vi "MainTypeClassic.vi"() -> ()   [LabVIEW 2014]
panel:
  in  "ButtonC":bool
  in  "ButtonB":bool
  in  "ButtonA":bool
  out "NowTime":timestamp
  out "MsgString":string
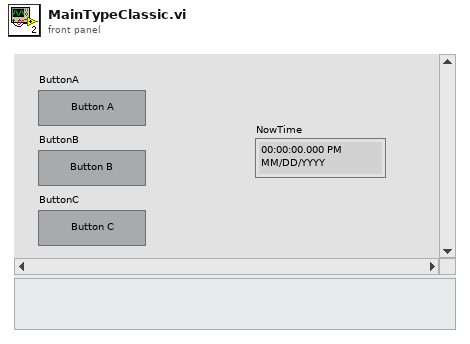
[diagram p1: front panel]
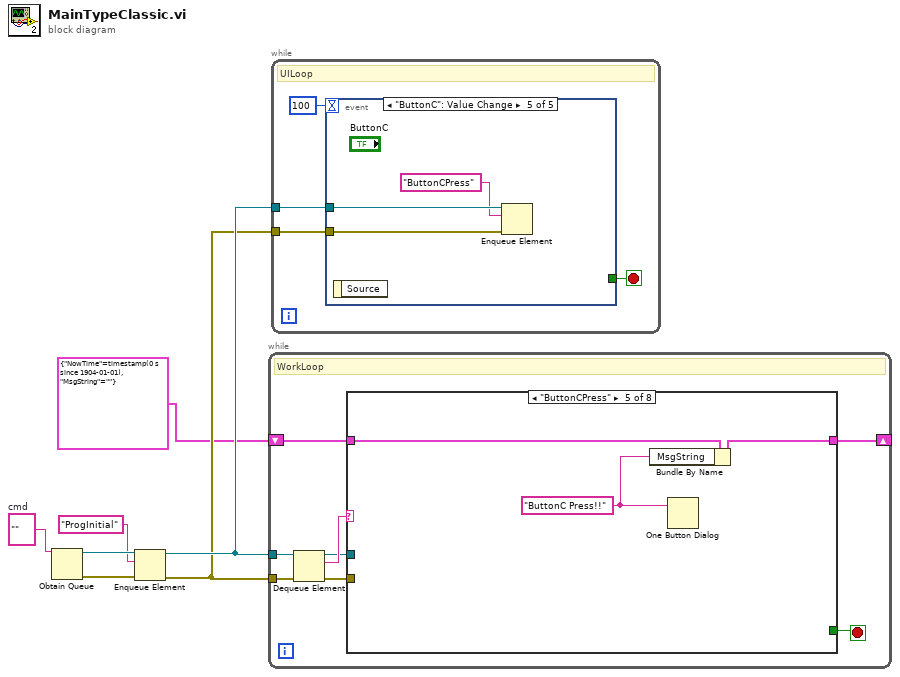
[diagram p0: block diagram]
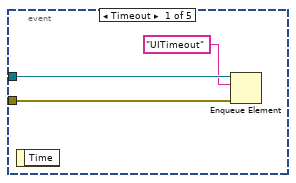
[diagram p2: hidden frame]
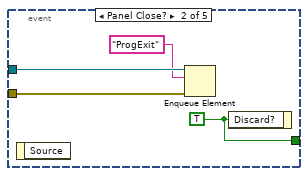
[diagram p3: hidden frame]
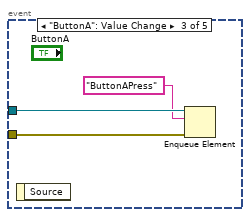
[diagram p4: hidden frame]
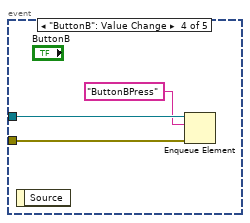
[diagram p5: hidden frame]
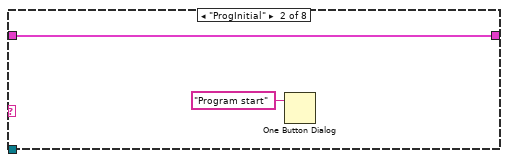
[diagram p7: hidden frame]
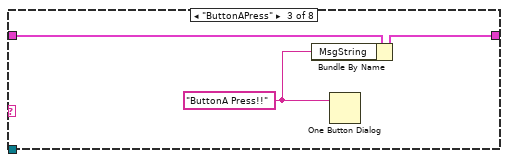
[diagram p8: hidden frame]
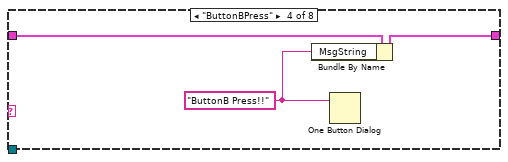
[diagram p9: hidden frame]
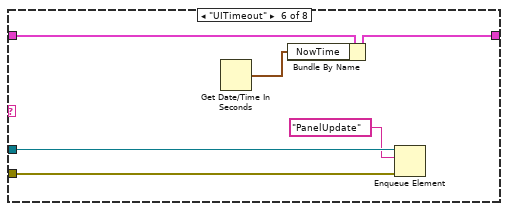
[diagram p10: hidden frame]
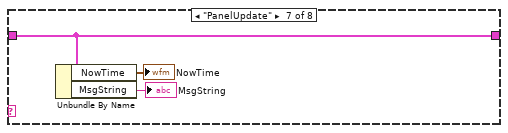
[diagram p11: hidden frame]
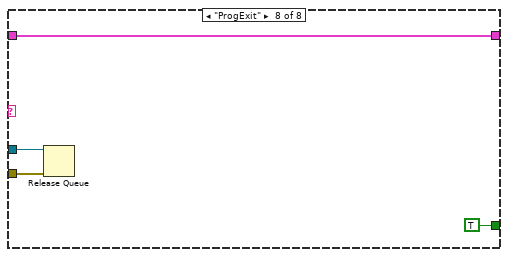
[diagram p12: hidden frame]
diagram:
  w5 = ""  # cmd
  n1 = Obtain Queue(element data type=w5) -> (queue out=w7:refnum<queue>, error out=w6:errorcluster)  [unwired: 4 in, 1 out]
  n2 = Enqueue Element(queue=w7, element="ProgInitial", error in (no error)=w6) -> (queue out=w3:refnum<queue>, error out=w2:errorcluster)  [unwired: 1 in, 1 out]
  n3 = while {
    tunnel: w3 -> [w15]
    tunnel: w2 -> [w14]
    shift-right: [w12] -> _
    shift-left: cluster{"NowTime":timestamp, "MsgString":string} {"NowTime"=timestamp(0 s since 1904-01-01), "MsgString"=""} -> [w11]
    stop <- w8 stop-if-true
    # "WorkLoop"
    n4 = Dequeue Element(queue=w15, error in (no error)=w14) -> (queue out=w10:refnum<queue>, element=w13:string, error out=w9:errorcluster)  [unwired: 1 in, 1 out]
    n5 = case shown="\"ButtonCPress\"" w13 {
      tunnel: [w16 w17 w20 w23 w26 w32 w36 w40] -> w12
      tunnel: w11 -> [w16 w17 w21 w24 w27 w33 w36 w40]
      tunnel: w10 -> [_ _ _ _ _ w30 _ w39]
      tunnel: w9 -> [_ _ _ _ _ w29 _ w38]
      tunnel: [_ _ _ _ _ _ _ TRUE ("Discard?")] -> w8
      frame Default {
      }
      frame "ProgInitial" {
        n6 = One Button Dialog(message="Program start") -> ()  [unwired: 1 in, 1 out]
      }
      frame "ButtonAPress" {
        w19 = "ButtonA Press!!" ("message")
        n7 = Bundle By Name(cluster=w21, "MsgString"=w19) -> (w20:cluster{"NowTime":timestamp, "MsgString":string})
        n8 = One Button Dialog(message=w19) -> ()  [unwired: 1 in, 1 out]
      }
      frame "ButtonBPress" {
        w22 = "ButtonB Press!!" ("message")
        n9 = Bundle By Name(cluster=w24, "MsgString"=w22) -> (w23:cluster{"NowTime":timestamp, "MsgString":string})
        n10 = One Button Dialog(message=w22) -> ()  [unwired: 1 in, 1 out]
      }
      frame "ButtonCPress" {
        w25 = "ButtonC Press!!" ("message")
        n11 = Bundle By Name(cluster=w27, "MsgString"=w25) -> (w26:cluster{"NowTime":timestamp, "MsgString":string})
        n12 = One Button Dialog(message=w25) -> ()  [unwired: 1 in, 1 out]
      }
      frame "UITimeout" {
        n13 = Get Date/Time In Seconds() -> (seconds since 1Jan1904=w31:timestamp)
        n14 = Bundle By Name(cluster=w33, "NowTime"=w31) -> (w32:cluster{"NowTime":timestamp, "MsgString":string})
        n15 = Enqueue Element(queue=w30, element="PanelUpdate", error in (no error)=w29) -> ()  [unwired: 1 in, 3 out]
      }
      frame "PanelUpdate" {
        n16 = Unbundle By Name(w36) -> ("NowTime"=→"NowTime":timestamp, "MsgString"=→"MsgString":string)
      }
      frame "ProgExit" {
        n17 = Release Queue(queue=w39, error in (no error)=w38) -> ()  [unwired: 1 in, 3 out]
      }
    }
  }
  n18 = while {
    tunnel: w3 -> [w43]
    tunnel: w2 -> [w42]
    stop <- w41 stop-if-true
    # "UILoop"
    n19 = event shown="[4] \"ButtonC\": Value Change" {
      selector: _ -> [_ _ _ _ _]
      dyn-events: _ -> [_ _ _ _ _]
      timeout: 100 -> [_ _ _ _ _]
      tunnel: w43 -> [w47 w51 w54 w57 w60]
      tunnel: w42 -> [w46 w50 w53 w56 w59]
      tunnel: [_ w49 _ _ _] -> w41
      event Timeout {
        n20 = event-data() -> ()  [unwired: 1 in, 1 out]
        n21 = Enqueue Element(queue=w47, element="UITimeout", error in (no error)=w46) -> ()  [unwired: 1 in, 3 out]
      }
      event Panel Close? {
        w49 = TRUE ("Discard?")
        n22 = event-data() -> ()  [unwired: 1 in, 1 out]
        n23 = Enqueue Element(queue=w51, element="ProgExit", error in (no error)=w50) -> ()  [unwired: 1 in, 3 out]
        n24 = event-data("Discard?"=w49) -> ()  [unwired: 1 in, 1 out]
      }
      event "ButtonA": Value Change {
        n25 = event-data() -> ()  [unwired: 1 in, 1 out]
        n26 = Enqueue Element(queue=w54, element="ButtonAPress", error in (no error)=w53) -> ()  [unwired: 1 in, 3 out]
      }
      event "ButtonB": Value Change {
        n27 = event-data() -> ()  [unwired: 1 in, 1 out]
        n28 = Enqueue Element(queue=w57, element="ButtonBPress", error in (no error)=w56) -> ()  [unwired: 1 in, 3 out]
      }
      event "ButtonC": Value Change {
        n29 = event-data() -> ()  [unwired: 1 in, 1 out]
        n30 = Enqueue Element(queue=w60, element="ButtonCPress", error in (no error)=w59) -> ()  [unwired: 1 in, 3 out]
      }
    }
  }
